vi "readSensor.vi"(8 "error in (no error)":errorcluster, 11 "PressureSensor in":refnum<class "PressureSensor.lvclass">) -> (0 "error out":errorcluster, 2 "Pressure Sensor 1":dbl format="%0.2f", 3 "PressureSensor out":refnum<class "PressureSensor.lvclass">)   [LabVIEW 2015, in "PressureSensor.lvclass"]
uses:
  PressureSensor.lvclass
  PressureSensor.lvclass/PressureSensor.ctl
  <vilib>/DAQmx/read.llb/DAQmx Read (Analog DBL 1Chan 1Samp).vi
  <vilib>/DAQmx/miscellaneous.llb/DAQmx Fill In Error Info.vi
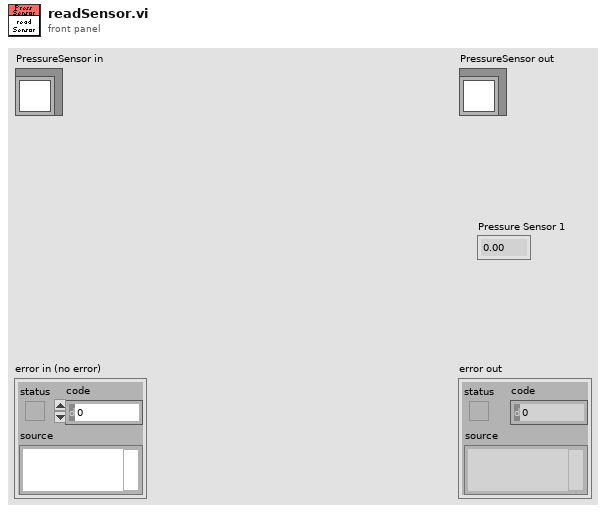
[diagram p1: front panel]
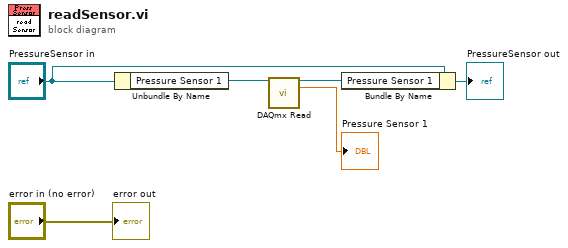
[diagram p0: block diagram]
diagram:
  n1 = Unbundle By Name("PressureSensor in") -> ("Pressure Sensor 1"=w5:refnum<k21>)
  n2 = call-poly <vilib>:"DAQmx Read.vi"("task/channels in"=w5) -> ("task out"=w1:refnum<k21>, "data"=→"Pressure Sensor 1":dbl)  [unwired: 12 in, 1 out]
  n3 = Bundle By Name(cluster="PressureSensor in", "Pressure Sensor 1"=w1) -> (→"PressureSensor out":refnum<class "PressureSensor.lvclass">)
  "error out" <- "error in (no error)"
